vi "ZCAN_ApplyAutoSend.vi"(7 "Eaable":bool, 8 "error in (no error)":errorcluster, 10 "DEVICE_HANDLE":u32, 11 "channelIdx":u32) -> (0 "error out":errorcluster, 3 "retunr":u32)   [LabVIEW 2020, in "zlgcan.lvlib"]
uses:
  zlgcan.lvlib
  bin/zlgcan_wrap.dll
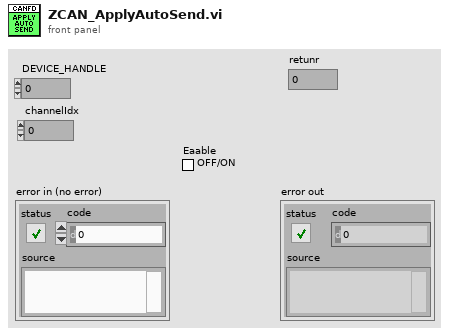
[diagram p1: front panel]
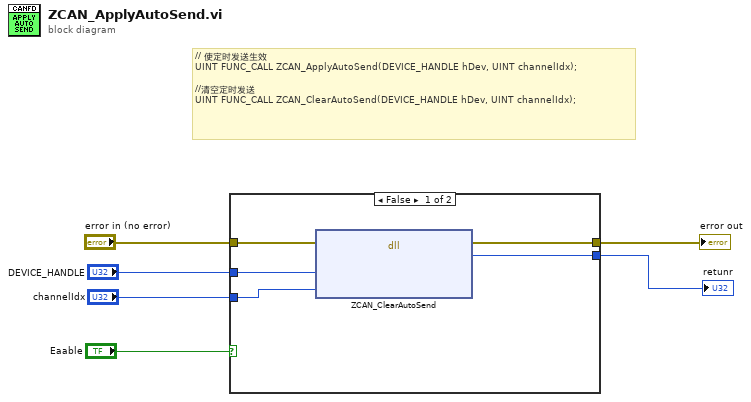
[diagram p0: block diagram]
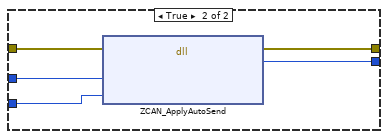
[diagram p2: hidden frame]
diagram:
  # "// 使定时发送生效\nUINT FUNC_CALL ZCAN_ApplyAutoSend(DEVICE_HANDLE hDev, UINT channelIdx);\n\n//清空定时发送\nUINT FUNC_CALL ZCAN_ClearAutoSend(DEVICE_HANDLE hDev, UINT channelIdx);"
  n1 = case shown="False" "Eaable" {
    tunnel: "DEVICE_HANDLE" -> [w8 w16]
    tunnel: "channelIdx" -> [w7 w15]
    tunnel: "error in (no error)" -> [w11 w14]
    tunnel: [w9 w13] -> w3
    tunnel: [w10 w12] -> w2
    frame False {
      n2 = dll-call lib="E:/Jabil tools/JabilTestLib/LV/ZLG_CANFD/bin/zlgcan_wrap.dll" fn="ZCAN_ClearAutoSend"(error in=w11, "DEVICE_HANDLE"=w8, "channelIdx"=w7) -> (error out=w10:errorcluster, "retunr"=w9:u32)  [unwired: 4 in, 1 out]
    }
    frame True {
      n3 = dll-call lib="E:/Jabil tools/JabilTestLib/LV/ZLG_CANFD/bin/zlgcan_wrap.dll" fn="ZCAN_ApplyAutoSend"(error in=w14, "DEVICE_HANDLE"=w16, "channelIdx"=w15) -> (error out=w12:errorcluster, "retunr"=w13:u32)  [unwired: 4 in, 1 out]
    }
  }
  "retunr" <- w3
  "error out" <- w2
